vi "GenNet Get Broadcast Name From Variant.vi"(10 "error in":errorcluster, 11 "Broadcast Data IN":variant) -> (2 "error out":errorcluster, 3 "Broadcast Data Out":variant, 5 "Broadcast Name":string)   [LabVIEW 2020, in "hse-gennet.lvlib"]
doc: "____\nHAMPEL SOFTWARE ENGINEERING v3.8.0 (2023-12-18 14:41)"
uses:
  hse-gennet.lvlib
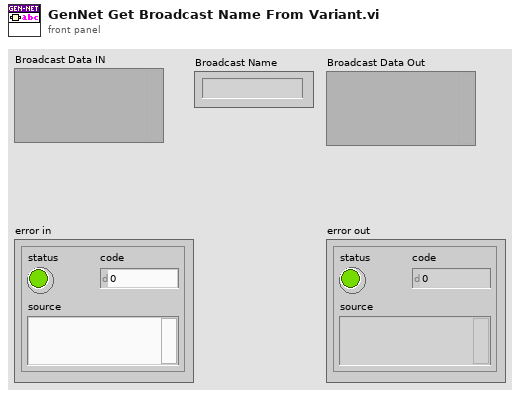
[diagram p1: front panel]
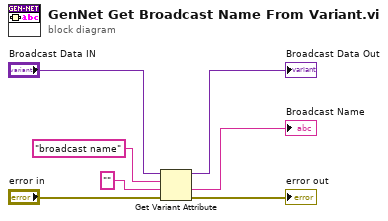
[diagram p0: block diagram]
diagram:
  n1 = Get Variant Attribute(Variant="Broadcast Data IN", name="broadcast name", default value (empty Variant)="", error in="error in") -> (duplicate Variant=→"Broadcast Data Out":variant, value=→"Broadcast Name":string, error out=→"error out":errorcluster)  [unwired: 1 out]
